vi "PID_control(SubVI).vi"(9 "Stop Button":bool, 10 "PID gains":T1={"proportional gain (Kc)"=1.0, "integral time (Ti, min)"=0.01, "derivative time (Td, min)"=0.0}, 11 "Numeric":i32) -> (0 "Numeric 2":dbl, 1 "Velocity":dbl, 2 "Numeric Control":i32, 3 "Waveform Chart":cluster{"Counter Value":i32, "Numeric":i32}(graph))   [LabVIEW 2017]
uses:
  <vilib>/addons/control/pid/pid.llb/PID (DBL).vi
  <vilib>/addons/control/pid/NI_PID_pid.lvlib
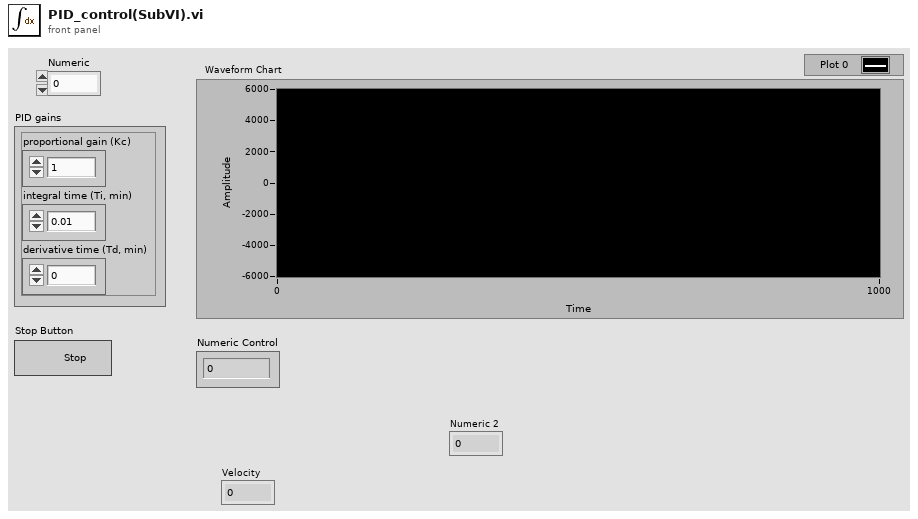
[diagram p1: front panel]
types:
  T1 = cluster{"proportional gain (Kc)":dbl, "integral time (Ti, min)":dbl, "derivative time (Td, min)":dbl}
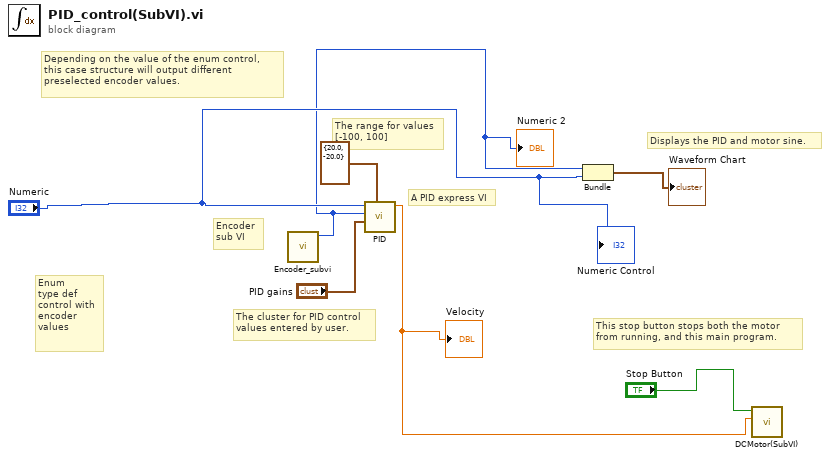
[diagram p0: block diagram]
diagram:
  # "Enum \ntype def\ncontrol with\nencoder\nvalues"
  # "This stop button stops both the motor \nfrom running, and this main program."
  # "Displays the PID and motor sine."
  # "Encoder \nsub VI"
  # "A PID express VI"
  # "The range for values\n[-100, 100]"
  # "The cluster for PID control\nvalues entered by user."
  # "Depending on the value of the enum control,\nthis case structure will output different \npreselected encoder values."
  n1 = call "Encoder_subvi.vi"() -> ("Counter Value"=w2:i32)  [unwired: 9 in, 2 out]
  "Numeric 2" <- w2
  n2 = call-poly <vilib>:"PID.vi"("output range"=cluster{"output high":dbl, "output low":dbl} {"output high"=20.0, "output low"=-20.0}, "PID gains"="PID gains", "process variable"=w2, "setpoint"="Numeric") -> ("output"=w1:dbl)  [unwired: 6 in, 1 out]
  "Velocity" <- w1
  n3 = Bundle("Counter Value"=w2, "Numeric"="Numeric") -> (→"Waveform Chart":cluster{"Counter Value":i32, "Numeric":i32})  [unwired: 1 in]
  n4 = call "DCMotor(SubVI).vi"("Duty Cycle (-100 to +100)"=w1, "Stop VI"="Stop Button") -> ()  [unwired: 9 in, 1 out]
  "Numeric Control" <- "Numeric"
